vi "Network_ApplyStatic.vi"(7 "DevInfo Original":T1={"Hostname"="", "IPAddress"="", "MAC"="", "SerialNum"="", "Model"="", "Status"="", "FW"="", "OSDesc"="", "ImgTitle"="", "ImgDesc"="", "ImgVer"="", "ImgID"="", "IP Address Request Mode"=1, "SubnetMask"="", "Gateway"="", "DNSServer"=""} {"IP Address Request Mode" items=["Static"=1, "DHCP/Link-Local"=2, "Link-Local Only"=4, "DHCP Only"=8]}, 8 "error in (no error)":errorcluster, 11 "DevInfo Modified":T1={"Hostname"="", "IPAddress"="", "MAC"="", "SerialNum"="", "Model"="", "Status"="", "FW"="", "OSDesc"="", "ImgTitle"="", "ImgDesc"="", "ImgVer"="", "ImgID"="", "IP Address Request Mode"=1, "SubnetMask"="", "Gateway"="", "DNSServer"=""} {"IP Address Request Mode" items=["Static"=1, "DHCP/Link-Local"=2, "Link-Local Only"=4, "DHCP Only"=8]}) -> (0 "error out":errorcluster)   [LabVIEW 2021]
uses:
  TypeDefs/DevInfo.ctl
  TypeDefs/TargetAccess.ctl
  <vilib>/nisyscfg/Save Changes (System).vi
  <vilib>/nisyscfg/Close (System).vi
  <resource>/objmgr/nisysapi.rc
  <vilib>/nisyscfg/nisyscfg.lvlib
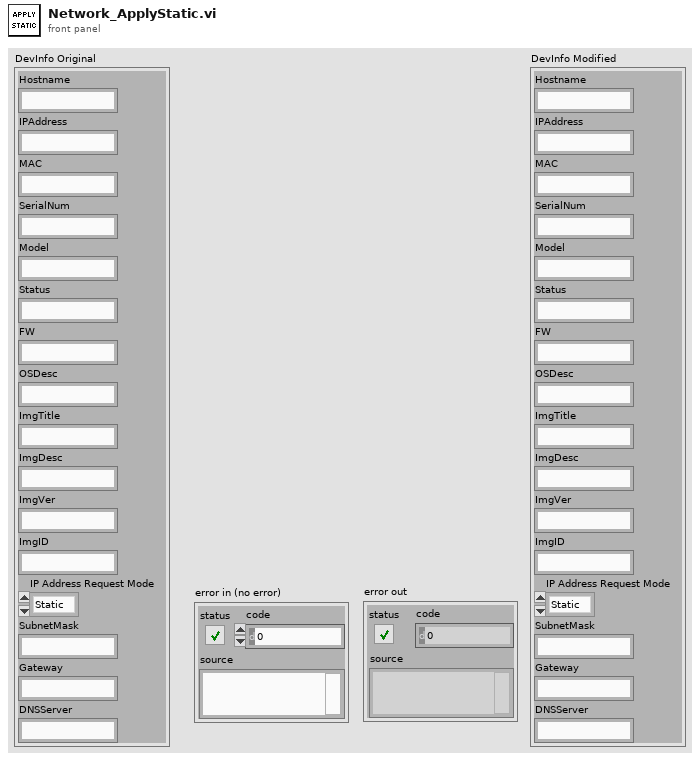
[diagram p1: front panel]
types:
  T1 = typedef "DevInfo.ctl" = cluster{"Hostname":string, "IPAddress":string, "MAC":string, "SerialNum":string, "Model":string, "Status":string, "FW":string, "OSDesc":string, "ImgTitle":string, "ImgDesc":string, "ImgVer":string, "ImgID":string, "IP Address Request Mode":i32, "SubnetMask":string, "Gateway":string, "DNSServer":string}
  T2 = typedef "TargetAccess.ctl" = enum16{"Read-Only", "Admin"}
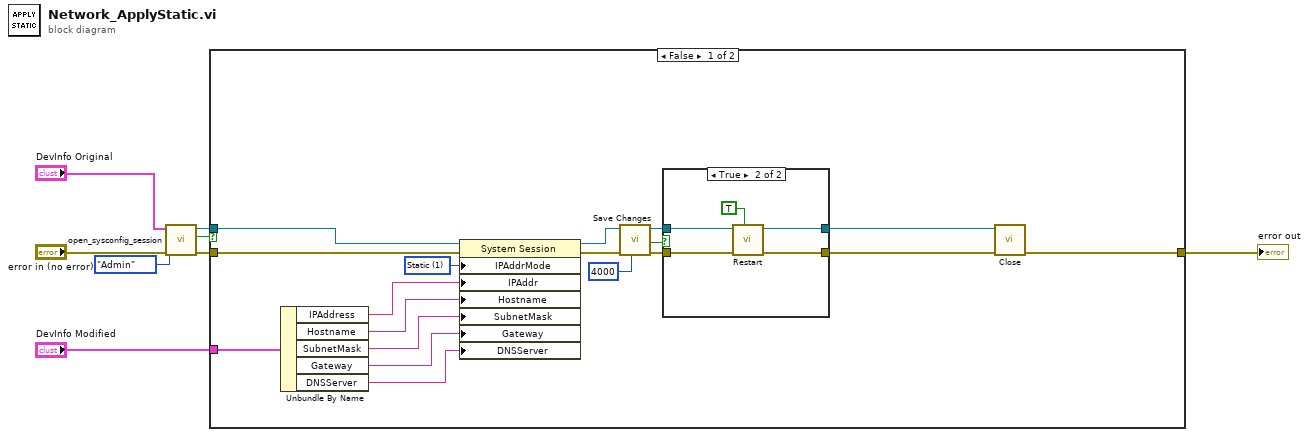
[diagram p0: block diagram]
diagram:
  n1 = call "open_sysconfig_session.vi"("error in (no error)"="error in (no error)", "Target Access"=TargetAccess."Admin", "DevInfo"="DevInfo Original") -> ("error out"=w5:errorcluster, "Cancelled"=w6:bool, "Session Out"=w4:refnum<k21>)  [unwired: 6 in]
  n2 = case shown="False" w6 {
    tunnel: w5 -> [w17 w34]
    tunnel: w4 -> [w18 _]
    tunnel: "DevInfo Modified" -> [w23 _]
    tunnel: [w19 w34] -> w2
    frame False {
      w14 = 1 items=["Static"=1, "DHCP/Link-Local"=2, "Link-Local Only"=4, "DHCP Only"=8] ("Primary NIC:IP Address Request Mode")
      n3 = Unbundle By Name(w23) -> ("IPAddress"=w13:string, "Hostname"=w12:string, "SubnetMask"=w11:string, "Gateway"=w10:string, "DNSServer"=w9:string)
      n4 = property class="System Session"(reference=w18, error in=w17, "IPAddrMode"=w14, "IPAddr"=w13, "Hostname"=w12, "SubnetMask"=w11, "Gateway"=w10, "DNSServer"=w9) -> (reference out=w15:refnum<k21>, error out=w16:errorcluster)
      n5 = call-poly <vilib>:"Save Changes.vi"("Remote Timeout (300,000 ms)"=u32 4000, "error in (no error)"=w16, "Session in"=w15) -> ("error out"=w25:errorcluster, "Changes Require Restart"=w24:bool, "Session out"=w26:refnum<k21>)  [unwired: 5 in, 1 out]
      n6 = case shown="True" w24 {
        tunnel: w25 -> [w27 w33]
        tunnel: [w27 w32] -> w21
        tunnel: w26 -> [w28 w31]
        tunnel: [w28 w30] -> w22
        frame False {
        }
        frame True {
          n7 = call <vilib>:"Restart.vi"("Wait Until Complete (T)"=TRUE ("wait until complete (T)"), "error in (no error)"=w33, "Session in"=w31) -> ("error out"=w32:errorcluster, "Session out"=w30:refnum<k21>)  [unwired: 6 in, 1 out]
        }
      }
      n8 = call-poly <vilib>:"Close.vi"("error in (no error)"=w21, "Session in"=w22) -> ("error out"=w19:errorcluster)  [unwired: 9 in]
    }
    frame True {
    }
  }
  "error out" <- w2
